vi "GETENUMdll.vi"(8 "error in (no error)":errorcluster, 10 "hEnum":string, 11 "iFlag":i32) -> (0 "error out":errorcluster, 3 "Outputs":T1)   [LabVIEW 2016]
doc: "subroutine GETENUMdll(iFlag, hEnum, iEnum, ierr, herr, hEnum_length, herr_length)\n\nTranslate a string of letters into an integer value that can be used in calls to ALLPROP0 to increase the speed\nof property calculations by eliminating string comparisons (which are time expensive in Fortran). This can be\ndone once at the beginning of a program for all properties that will be used, and stored for use as needed later.\nThe input strings possible are described in subroutines ALLPROPSdll() and GETUNITdll().\n\nINPUTS:\niFlag -- Flag to specify which type of enumerated value to return\n 0 Check all strings possible.\n 1 Check strings for property units only (e.g., SI, English, etc.).\n 2 Check property strings and those in #3 only.\n 3 Check property strings only that are not functions of T and D. (for example, the\n critical point, acentric factor, limits of the EOS, etc.)\nhEnum -- The string that will be used to return the enumerated value. Only uppercase letters are allowed to decrease the time required to process the values.\n\nOUTPUTS:\niEnum -- The enumerated value that matches the string sent in hEnum.\nierr -- Error flag\nherr -- Error string (character*255)\nhEnum_length -- length of variable hEnum (default: 255)\nherr_length -- length of variable herr (default: 255)"
uses:
  REFPROP.DLL
panel:
  # "REFPROP-GETENUMdll.vi"
  # "void  GETENUMdll(int32_t *iFlag, CStr hEnum, int32_t *iEnum, int32_t *ierr, CStr herr, int32_t hEnum_length, int32_t *herr_length);"
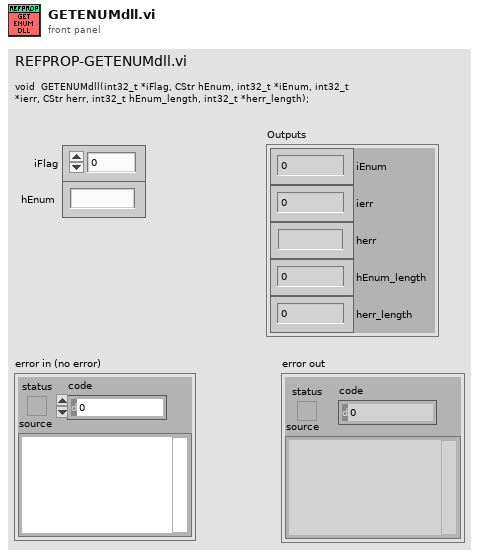
[diagram p1: front panel]
types:
  T1 = cluster{"iEnum":i32, "ierr":i32, "herr":string, "hEnum_length":i32, "herr_length":i32}
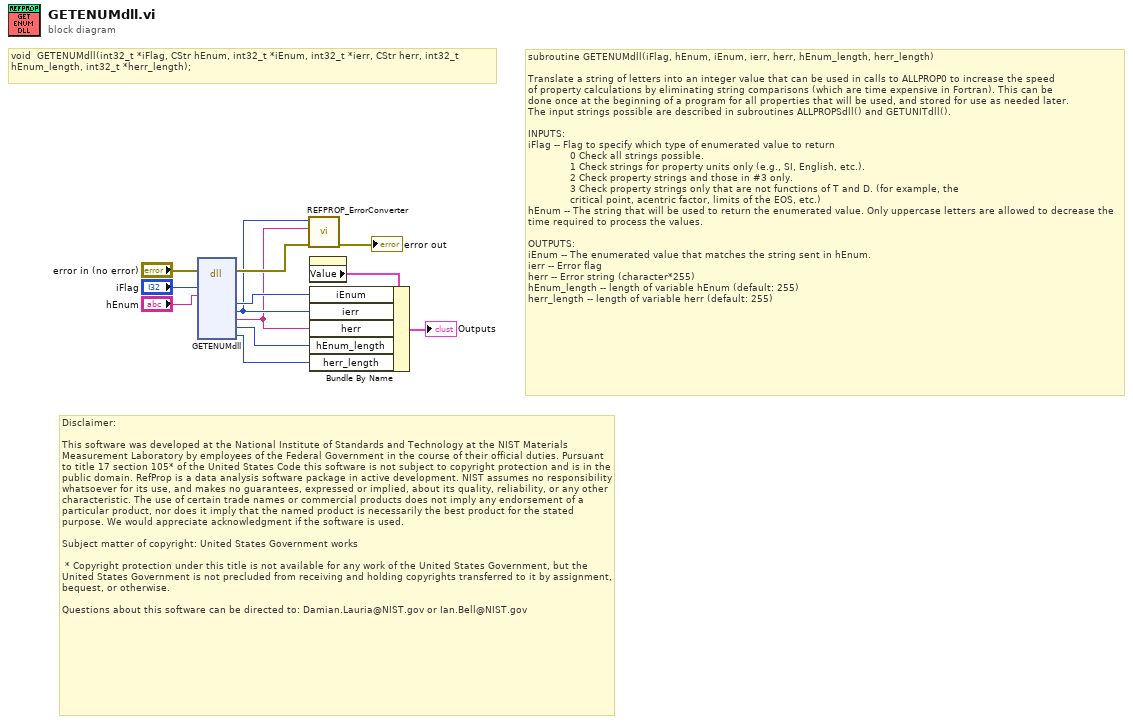
[diagram p0: block diagram]
diagram:
  # "void  GETENUMdll(int32_t *iFlag, CStr hEnum, int32_t *iEnum, int32_t *ierr, CStr herr, int32_t hEnum_length, int32_t *herr_length);"
  # "Disclaimer:\n\nThis software was developed at the National Institute of Standards and Technology at the NIST Materials Measurement Laboratory by employees of the Federal Government in the course of their official duties. Pursuant to title 17 section 105* of the United States Code this software is not subject to copyright protection and is in the public domain. RefProp is a data analysis software package in active development. NIST assumes no responsibility whatsoever for its use, and makes no guarantees, expressed or implied, about its quality, reliability, or any other characteristic. The use of certain trade names or commercial products does not imply any endorsement of a particular product, nor does it imply that the named product is necessarily the best product for the stated purpose. We would appreciate acknowledgment if the software is used.\n \nSubject matter of copyright: United States Government works\n  \n * Copyright protection under this title is not available for any work of the United States Government, but the United States Government is not precluded from receiving and holding copyrights transferred to it by assignment, bequest, or otherwise.\n\nQuestions about this software can be directed to: Damian.Lauria@NIST.gov or Ian.Bell@NIST.gov"
  # "subroutine GETENUMdll(iFlag, hEnum, iEnum, ierr, herr, hEnum_length, herr_length)\n\nTranslate a string of letters into an integer value that can be used in calls to ALLPROP0 to increase the speed\nof property calculations by eliminating string comparisons (which are time expensive in Fortran). This can be\ndone once at the beginning of a program for all properties that will be used, and stored for use as needed later.\nThe input strings possible are described in subroutines ALLPROPSdll() and GETUNITdll().\n\nINPUTS:\niFlag -- Flag to specify which type of enumerated value to return\n              0 Check all strings possible.\n              1 Check strings for property units only (e.g., SI, English, etc.).\n              2 Check property strings and those in #3 only.\n              3 Check property strings only that are not functions of T and D. (for example, the\n              critical point, acentric factor, limits of the EOS, etc.)\nhEnum -- The string that will be used to return the enumerated value. Only uppercase letters are allowed to decrease the time required to process the values.\n\nOUTPUTS:\niEnum -- The enumerated value that matches the string sent in hEnum.\nierr -- Error flag\nherr -- Error string (character*255)\nhEnum_length -- length of variable hEnum (default: 255)\nherr_length -- length of variable herr (default: 255)"
  n1 = dll-call lib="S:/009 - Testing/02 - Performance Testing/REFPROP/REFPROP.*" fn="GETENUMdll"(error in="error in (no error)", "iFlag"="iFlag", "hEnum"="hEnum") -> (error out=w12:errorcluster, "iEnum"=w6:i32, "ierr"=w5:i32, "herr"=w4:string, "hEnum_length"=w3:i32, "herr_length"=w2:i32)  [unwired: 10 in, 1 out]
  n2 = call "REFPROP_ErrorConverter.vi"("error in (no error)"=w12, "Error Message"=w4, "Error Code"=w5) -> ("error out"=→"error out":errorcluster)  [unwired: 8 in]
  n3 = property on="Outputs" class="Clust (strict)"() -> ("Value"=w7:T1)  [unwired: 2 in, 2 out]
  n4 = Bundle By Name(cluster=w7, "iEnum"=w6, "ierr"=w5, "herr"=w4, "hEnum_length"=w3, "herr_length"=w2) -> (→"Outputs":T1)
